vi "Get Page VI.vi"(8 "error in":errorcluster, 9 "GUID":string, 10 "item ref":T1 format="%.0x", 11 "System Explorer Dispatcher Implementation in":refnum<class "System Explorer Dispatcher.lvclass">) -> (0 "error out":errorcluster, 2 "page reference":refnum<vi>, 3 "System Explorer Dispatcher Implementation out":refnum<class "System Explorer Dispatcher.lvclass">)   [LabVIEW 2020, in "Ballard MIL-STD-1553 System Explorer.lvlib" / "Implementation.lvlib" / "System Explorer Dispatcher.lvclass"]
uses:
  System Explorer Dispatcher.lvclass
  Implementation.lvlib
  Scripting/Constants.vi
  Scripting/Ballard MIL-STD-1553 Scripting.lvlib
  System Explorer/Pages/Configuration Files.vi
  System Explorer/Pages/Parameter.vi
  System Explorer/Pages/Command Channel.vi
  System Explorer/Pages/Status.vi
  System Explorer/Pages/Receive Time.vi
  <vilib>/NI VeriStand/Custom Device API/Custom Device Item Ref.ctl
  <vilib>/NI VeriStand/Custom Device API/Custom Device API.lvlib
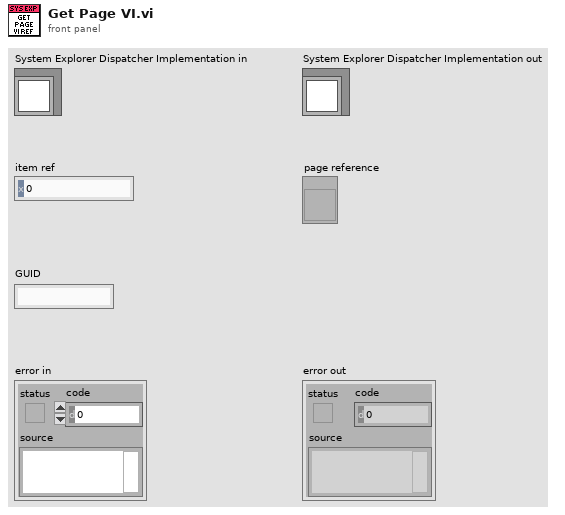
[diagram p1: front panel]
types:
  T1 = typedef "Custom Device API.lvlib/Custom Device Item Ref.ctl" = u64
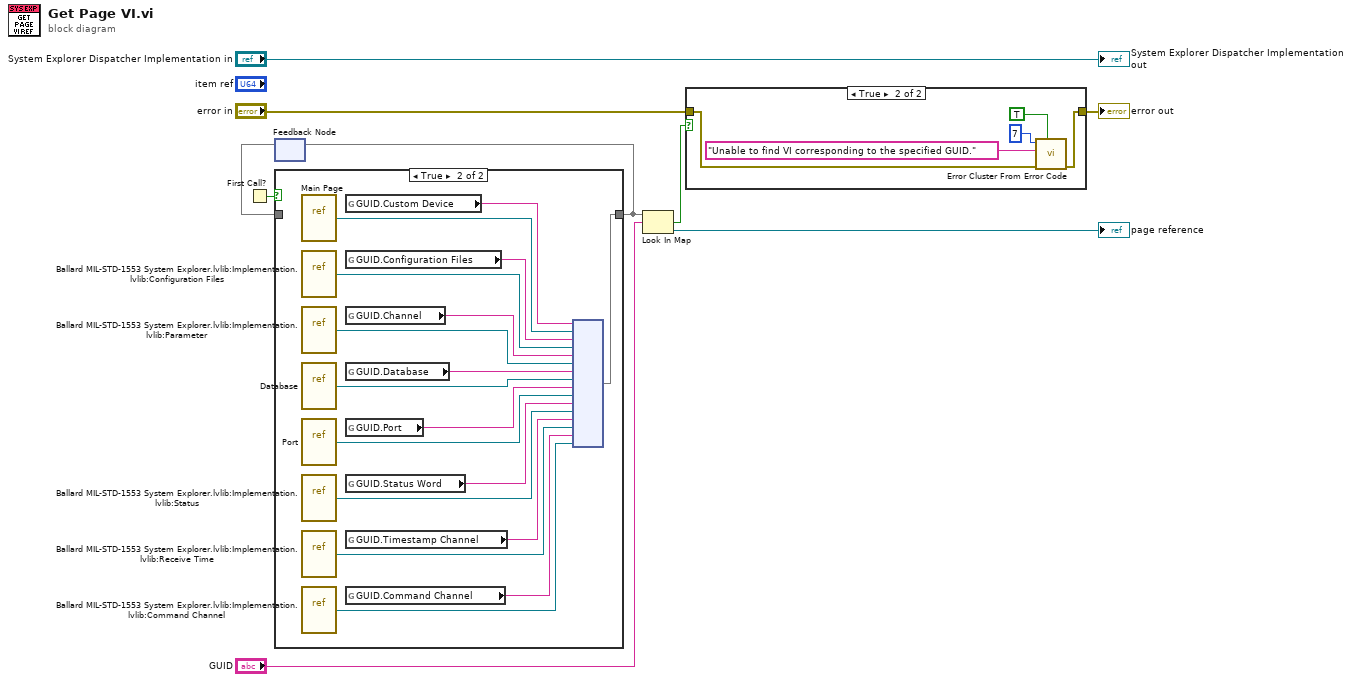
[diagram p0: block diagram]
diagram:
  n1 = First Call?() -> (First Call?: T/F=w8:bool)
  n2 = feedback #1() -> (w7:map{string, refnum<vi>})  [unwired: 1 in]
  n3 = case shown="True" w8 {
    tunnel: [w10 w27] -> w6
    tunnel: w7 -> [w10 _]
    frame False {
    }
    frame True {
      n4 = vi-ref "Main Page.vi"() -> (w26:refnum<vi>)
      n5 = vi-ref "Ballard MIL-STD-1553 System Explorer.lvlib:Implementation.lvlib:Configuration Files.vi"() -> (w24:refnum<vi>)
      n6 = vi-ref "Ballard MIL-STD-1553 System Explorer.lvlib:Implementation.lvlib:Parameter.vi"() -> (w21:refnum<vi>)
      n7 = vi-ref "Database.vi"() -> (w19:refnum<vi>)
      n8 = vi-ref "Port.vi"() -> (w17:refnum<vi>)
      n9 = vi-ref "Ballard MIL-STD-1553 System Explorer.lvlib:Implementation.lvlib:Status.vi"() -> (w15:refnum<vi>)
      n10 = vi-ref "Ballard MIL-STD-1553 System Explorer.lvlib:Implementation.lvlib:Receive Time.vi"() -> (w13:refnum<vi>)
      n11 = vi-ref "Ballard MIL-STD-1553 System Explorer.lvlib:Implementation.lvlib:Command Channel.vi"() -> (w11:refnum<vi>)
      n12 = global read "Constants.vi" "GUID.Custom Device"() -> (w25:string)
      n13 = global read "Constants.vi" "GUID.Configuration Files"() -> (w23:string)
      n14 = global read "Constants.vi" "GUID.Channel"() -> (w22:string)
      n15 = global read "Constants.vi" "GUID.Database"() -> (w20:string)
      n16 = global read "Constants.vi" "GUID.Port"() -> (w18:string)
      n17 = global read "Constants.vi" "GUID.Status Word"() -> (w16:string)
      n18 = global read "Constants.vi" "GUID.Timestamp Channel"() -> (w14:string)
      n19 = global read "Constants.vi" "GUID.Command Channel"() -> (w12:string)
      n20 = node(w25, w26, w23, w24, w22, w21, w20, w19, w18, w17, w16, w15, w14, w13, w12, w11) -> (w27:map{string, refnum<vi>})
    }
  }
  n21 = feedback-in #1(w6) -> ()
  n22 = Look In Map(map=w6, key="GUID") -> (key not found?=w4:bool, value=→"page reference":refnum<vi>)  [unwired: 1 in]
  n23 = case shown="True" w4 {
    tunnel: [w28 w30] -> w3
    tunnel: "error in" -> [w28 w29]
    frame False {
    }
    frame True {
      n24 = call <vilib>:"Error Cluster From Error Code.vi"("show call chain? (False)"=TRUE, "error in (no error)"=w29, "error message (\"\")"="Unable to find VI corresponding to the specified GUID." ("error message (\"\")"), "error code (0)"=7) -> ("error out"=w30:errorcluster)  [unwired: 5 in]
    }
  }
  "error out" <- w3
  "System Explorer Dispatcher Implementation out" <- "System Explorer Dispatcher Implementation in"
